vi "magic.vi"(8 "error in":errorcluster, 11 "payload":string) -> (0 "error out":errorcluster, 3 "body":string)   [LabVIEW 2020]
uses:
  <vilib>/httpClient/POSTBuffer.vi
  <vilib>/httpClient/PUTBuffer.vi
  <vilib>/httpClient/LabVIEWHTTPClient.lvlib
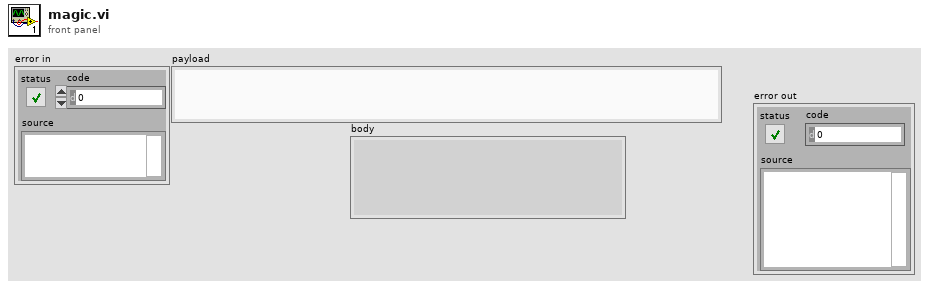
[diagram p1: front panel]
types:
  T1 = cluster{"method":string, "url":string, "headers":string}
  T2 = typedef "LabVIEWHTTPClient.lvlib/ClientHandle.ctl" = refnum<k1>
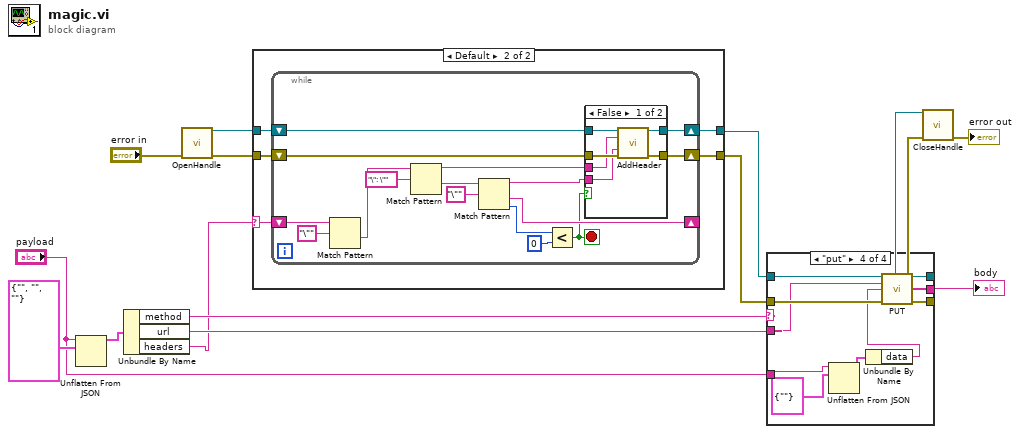
[diagram p0: block diagram]
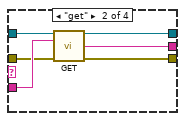
[diagram p5: hidden frame]
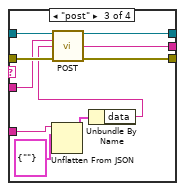
[diagram p6: hidden frame]
diagram:
  n1 = Unflatten From JSON(JSON string="payload", type and defaults=T1 {"method"="", "url"="", "headers"=""}) -> (value=w2:T1)  [unwired: 5 in, 1 out]
  n2 = Unbundle By Name(w2) -> ("method"=w11:string, "url"=w10:string, "headers"=w3:string)
  n3 = call <vilib>:"OpenHandle.vi"("error in (no error)"="error in") -> ("client handle out"=w7:T2, "error out"=w6:errorcluster)  [unwired: 13 in]
  n4 = case shown="Default" w3 {
    selector: w3 -> [_ w18]
    tunnel: [w17 w22] -> w13
    tunnel: w7 -> [w17 w21]
    tunnel: w6 -> [w16 w20]
    tunnel: [w16 w19] -> w5
    frame "" {
    }
    frame Default {
      n5 = while {
        shift-right: [w25] -> _
        shift-left: w18 -> [w37]
        shift-right: [w34] -> w22
        shift-left: w21 -> [w35]
        shift-right: [w32] -> w19
        shift-left: w20 -> [w33]
        stop <- w23 stop-if-true
        n6 = Match Pattern(string=w37, regular expression="\"") -> (after substring=w30:string)  [unwired: 1 in, 3 out]
        n7 = Match Pattern(string=w30, regular expression="\": \"") -> (before substring=w28:string, after substring=w27:string)  [unwired: 1 in, 2 out]
        n8 = Match Pattern(string=w27, regular expression="\"") -> (before substring=w26:string, after substring=w25:string, offset past match=w24:i32)  [unwired: 1 in, 1 out]
        n9 = Less?(x=w24, y=0) -> (x < y?=w23:bool)
        n10 = case shown="False" w23 {
          tunnel: w35 -> [w44 w45]
          tunnel: [w43 w45] -> w34
          tunnel: w33 -> [w42 w46]
          tunnel: [w41 w46] -> w32
          tunnel: w28 -> [w40 _]
          tunnel: w26 -> [w39 _]
          frame False {
            n11 = call <vilib>:"AddHeader.vi"("client handle"=w44, "header"=w40, "value"=w39, "error in (no error)"=w42) -> ("client handle out"=w43:T2, "error out"=w41:errorcluster)  [unwired: 10 in]
          }
          frame True {
          }
        }
      }
    }
  }
  n12 = case shown="\"put\"" w11 {
    tunnel: [w47 w54 w64 w74] -> w14
    tunnel: w10 -> [_ w53 w59 w70]
    tunnel: [_ w52 w63 w69] -> w9
    tunnel: w5 -> [w48 w51 w62 w73]
    tunnel: [w48 w50 w61 w72] -> w15
    tunnel: w13 -> [w47 w49 w60 w71]
    tunnel: "payload" -> [_ _ w57 w68]
    frame Default {
    }
    frame "get" {
      n13 = call <vilib>:"GET.vi"("client handle"=w49, "url"=w53, "error in (no error)"=w51) -> ("client handle out"=w54:T2, "body"=w52:string, "error out"=w50:errorcluster)  [unwired: 9 in, 1 out]
    }
    frame "post" {
      n14 = Unflatten From JSON(JSON string=w57, type and defaults=cluster{"data":string} {"data"=""}) -> (value=w56:cluster{"data":string})  [unwired: 5 in, 1 out]
      n15 = Unbundle By Name(w56) -> ("data"=w58:string)
      n16 = call-poly <vilib>:"POST.vi"("client handle"=w60, "url"=w59, "buffer"=w58, "error in (no error)"=w62) -> ("client handle out"=w64:T2, "body"=w63:string, "error out"=w61:errorcluster)  [unwired: 8 in, 1 out]
    }
    frame "put" {
      n17 = Unflatten From JSON(JSON string=w68, type and defaults=cluster{"data":string} {"data"=""}) -> (value=w67:cluster{"data":string})  [unwired: 5 in, 1 out]
      n18 = Unbundle By Name(w67) -> ("data"=w66:string)
      n19 = call-poly <vilib>:"PUT.vi"("client handle"=w71, "url"=w70, "buffer"=w66, "error in (no error)"=w73) -> ("client handle out"=w74:T2, "body"=w69:string, "error out"=w72:errorcluster)  [unwired: 8 in, 1 out]
    }
  }
  "body" <- w9
  n20 = call <vilib>:"CloseHandle.vi"("client handle"=w14, "error in (no error)"=w15) -> ("error out"=→"error out":errorcluster)  [unwired: 13 in]
